vi "UI.vi"(8 "ErrorIn":errorcluster, 11 "QueuesIn":T1) -> (0 "ErrorOut":errorcluster, 3 "QueuesOut":T1)   [LabVIEW 2019]
uses:
  utilities/AQueues.ctl
  AmasterVIs/ACommand.ctl
  analyzeAccelerationDataVIs/AnalyzedVibrationsData.ctl
  analyzeAccelerationDataVIs/AccelerationDataFrames.ctl
  analyzeAccelerationDataVIs/calculateFaultIndicatorsVIs/FaultDetections.ctl
  analyzeAccelerationDataVIs/calculateFaultIndicatorsVIs/ParameterFaultDetection.ctl
  analyzeAccelerationDataVIs/calculateFaultIndicatorsVIs/FaultParameter.ctl
  analyzeAccelerationDataVIs/calculateFaultIndicatorsVIs/FrequencyFaultDetection.ctl
  analyzeAccelerationDataVIs/calculateFaultIndicatorsVIs/OrdersFaultDetection.ctl
  TDMSmanagerVIs/TDMSAnalyzerData.ctl
  TDMSmanagerVIs/TDMSAnalyzerDataType.ctl
  UIVIs/UIState.ctl
  <vilib>/dex/Stream Element Allocation Mode.ctl
  VibrationDiagnosisDesktopApp/mainVIs/communicateWithAnalyzerVIs/ReceiverData.ctl
  VibrationDiagnosisDesktopApp/mainVIs/communicateWithAnalyzerVIs/ReceiverDataType.ctl
  UIVIs/UIOutputFGVAction.ctl
  <vilib>/myRIO/Instrument Drivers/Onboard IO/DIO/typedefs/DIO Reference.ctl
  <vilib>/myRIO/Common/Instrument Driver Framework/Utilities/typedefs/myRIO Generic Hardware Reference.ctl
  <vilib>/myRIO/Common/Instrument Driver Framework/Utilities/typedefs/Hardware Version Enum.ctl
  <vilib>/myRIO/Common/Instrument Driver Framework/Utilities/typedefs/myRIO v1.0 Reference.ctl
  <vilib>/myRIO/Common/Instrument Driver Framework/Utilities/typedefs/Generic FPGA Reference.ctl
  <vilib>/myRIO/Common/Instrument Driver Framework/myRIO v1.0/DIO/typedefs/DIO Channels List.ctl
  <vilib>/myRIO/Common/Instrument Driver Framework/myRIO v1.0/DIO/typedefs/DIO Channels Enum.ctl
  <vilib>/userdefined/High Color/nirio_resource_hc.ctl
  VibrationDiagnosisDesktopApp/mainVIs/communicateWithAnalyzerVIs/SenderData.ctl
  VibrationDiagnosisDesktopApp/mainVIs/communicateWithAnalyzerVIs/SenderDataType.ctl
  utilities/FGVAction.ctl
  VibrationDiagnosisDesktopApp/mainVIs/DialogsVIs/AnalysisSettings.ctl
  analyzeAccelerationDataVIs/calculateFaultIndicatorsVIs/Thresholds.ctl
  aquireAccelerationDataVIs/Accelerometer.ctl
  <vilib>/myRIO/Common/Instrument Driver Framework/Utilities/vis/Is FPGA Ref Available.vi
  <vilib>/myRIO/Common/Instrument Driver Framework/myRIO v1.0/DIO/vis/myRIO v1.1 Open Throughput DIO.vi
  <vilib>/myRIO/Instrument Drivers/Onboard IO/DIO/vis/Read.vi
  <vilib>/myRIO/Instrument Drivers/Onboard IO/DIO/vis/Write.vi
  <vilib>/myRIO/Common/Instrument Driver Framework/Utilities/vis/Validate Channels.vi
  <vilib>/myRIO/Common/Instrument Driver Framework/myRIO v1.0/DIO/vis/myRIO v1.0 Reserve DIO.vi
  <vilib>/myRIO/Common/Instrument Driver Framework/myRIO v1.0/Resource Manager/vis/myRIO v1.0 Reserve Channel List.vi
  <vilib>/myRIO/Common/Instrument Driver Framework/myRIO v1.0/DIO/vis/myRIO v1.0 Build MUX Configuration DIO.vi
  <vilib>/myRIO/Common/Instrument Driver Framework/myRIO v1.0/Resource Manager/vis/myRIO v1.0 Reserve Channel.vi
  <vilib>/myRIO/Common/Instrument Driver Framework/myRIO v1.0/Resource Manager/vis/myRIO v1.0 Unreserve Channel.vi
  <vilib>/myRIO/Common/Instrument Driver Framework/myRIO v1.0/Resource Manager/vis/myRIO v1.0 Create Configuration List.vi
  <vilib>/myRIO/Common/Instrument Driver Framework/myRIO v1.0/Resource Manager/vis/myRIO v1.0 Build Mutex Name.vi
  <vilib>/Utility/VariantDataType/GetNumericInfo.vi
  <vilib>/Utility/error.llb/Error Cluster From Error Code.vi
  <vilib>/myRIO/Common/Instrument Driver Framework/myRIO v1.0/myRIO v1.1 Open Throughput.vi
  <vilib>/myRIO/Common/Instrument Driver Framework/Utilities/vis/IO Manager.vi
  <vilib>/myRIO/Common/Instrument Driver Framework/Utilities/vis/Configuration Manager.vi
  <vilib>/myRIO/Common/Instrument Driver Framework/myRIO v1.0/Resource Manager/vis/myRIO v1.0 Configure IO.vi
  <vilib>/myRIO/Common/Instrument Driver Framework/myRIO v1.0/myRIO v1.0 Close.vi
  <vilib>/myRIO/Common/Instrument Driver Framework/myRIO v1.0/DIO/vis/myRIO v1.0 Read DIO.vi
  <vilib>/myRIO/Common/Instrument Driver Framework/myRIO v1.0/DIO/vis/myRIO v1.0 Write DIO.vi
  <vilib>/myRIO/Express VI/Onboard Devices/Button/Button Express VI.xnode
  <vilib>/myRIO/Instrument Drivers/Onboard IO/DIO/vis/myRIO DIO Open.xnode
  <vilib>/myRIO/Express VI/Onboard Devices/LED/LED Express VI.xnode
  <vilib>/myRIO/Instrument Drivers/Onboard IO/DIO/DIO.lvlib
panel:
  in  "Restart":bool
  in  "OutputConnected":bool
  in  "InputConnected":bool
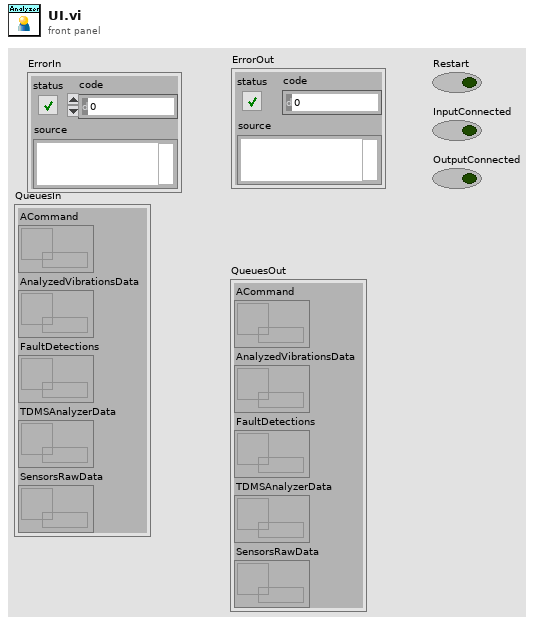
[diagram p1: front panel]
types:
  T1 = typedef "AQueues.ctl" = cluster{"ACommand":refnum<queue>, "AnalyzedVibrationsData":refnum<queue>, "FaultDetections":refnum<queue>, "TDMSAnalyzerData":refnum<queue>, "SensorsRawData":refnum<queue>}
  T2 = typedef "UIState.ctl" = enum16{"Connect", "Communicate", "Disconnect"}
  T3 = typedef "ACommand.ctl" = enum16{"None", "Start", "Stop", "Restart", "SendFilesData", "DeleteAllData", "ButtonClicked"}
  T4 = typedef "DIO.lvlib/DIO Reference.ctl" = cluster{"myRIO Reference":T5, "DIO Channels List":T9}
  T5 = typedef "myRIO Generic Hardware Reference.ctl" = cluster{"myRIO Model":T6, "myRIO Hardware Reference":T7}
  T6 = typedef "Hardware Version Enum.ctl" = enum16{"Unknown", "myRIO-1900", "myRIO-1950", "roboRIO", "NI ELVIS RIO CM", "ELVIS III"}
  T7 = typedef "myRIO v1.0 Reference.ctl" = cluster{"Generic FPGA Reference":T8, "Allow multiple opens":bool}
  T8 = typedef "Generic FPGA Reference.ctl" = refnum<k20>
  T9 = typedef "DIO Channels List.ctl" = T10[]
  T10 = typedef "DIO Channels Enum.ctl" = enum16{"Not Connected", "C/DIO0", "C/DIO1", "C/DIO2", "C/DIO3", "C/DIO4", "C/DIO5", "C/DIO6", "C/DIO7", "A/DIO0", "A/DIO1", "A/DIO2", "A/DIO3", "A/DIO4", "A/DIO5", "A/DIO6", "A/DIO7", "A/DIO8", "A/DIO9", "A/DIO10", "A/DIO11", "A/DIO12", "A/DIO13", "A/DIO14", "A/DIO15", "A/DIO16", "A/DIO17", "A/DIO18", "A/DIO19", "B/DIO0", "B/DIO1", "B/DIO2", "B/DIO3", "B/DIO4", "B/DIO5", "B/DIO6", "B/DIO7", "B/DIO8", "B/DIO9", "B/DIO10", "B/DIO11", "B/DIO12", "B/DIO13", "B/DIO14", "B/DIO15", "B/DIO16", "B/DIO17", "B/DIO18", "B/DIO19", "LED0", "LED1", "LED2", "LED3", "Button0", "DIO/DIO0", "DIO/DIO1", "DIO/DIO2", "DIO/DIO3", "DIO/DIO4", "DIO/DIO5", "DIO/DIO6", "DIO/DIO7", "DIO/DIO8", "DIO/DIO9", "SPI/CS0", "SPI/CS1", "SPI/CS2", "SPI/CS3", "LED RADIO (Green)", "LED RADIO (Red)", "LED COMM (Green)", "LED COMM (Red)", "LED MODE (Green)", "LED MODE (Red)"}
  T11 = typedef "nirio_resource_hc.ctl" = tag
  T12 = typedef "ReceiverData.ctl" = cluster{"ReceiverDataType":T13, "Data":string}
  T13 = typedef "ReceiverDataType.ctl" = enum16{"UIOutput", "AnalyzedVibrationsData", "TDMSFiles"}
  T14 = typedef "UIOutputFGVAction.ctl" = enum16{"Read", "Write", "CheckUpdate", "SetUpdated"}
  T15 = typedef "Stream Element Allocation Mode.ctl" = u32
  T16 = typedef "AnalyzerSettings.ctl" = cluster{"Create NS Timeout Code":i32, "Destroy NS Timeout Code":i32, "All threads":T17[], "Connected to app?":bool, "AnalysisSettings":T18}
  T17 = typedef "AThreads.ctl" = enum16{"UI", "analyzeAccelerationData", "aquireAccelerationData", "communicateWebServices", "TDMSmanager", "aquireTachoSignal"}
  T18 = typedef "AnalysisSettings.ctl" = cluster{"Fault Thresholds":T19, "Analysis series name":string, "Save data analysis?":bool, "Band size":i32, "OrderAnalysis?":bool, "Accelerometer":T21, "fs [Hz]":dbl, "Pulse per revolution":u16}
  T19 = typedef "Thresholds.ctl" = cluster{"Parameters labels":T20[], "Parameters thresholds":dbl[], "Freqs and thresholds":dbl[][], "Orders and thresholds":dbl[][]}
  T20 = typedef "FaultParameter.ctl" = enum16{"Kurtosis", "RMS", "Crest factor"}
  T21 = typedef "Accelerometer.ctl" = enum16{"None", "MPU6050", "MMA7351"}
  T22 = typedef "AnalyzedVibrationsData.ctl" = cluster{"AccelerationDataFrames":T23, "Fault detections":T24, "Order Power Spectra":cluster{"order 0":dbl, "delta order":dbl, "magnitude":dbl[]}[], "Tacho signal":waveform(dbl), "Rotational speed [RPM]":dbl}
  T23 = typedef "AccelerationDataFrames.ctl" = cluster{"AccelerationData":waveform(dbl)[], "Amplitudes":cluster{"f0":dbl, "df":dbl, "real part":dbl[]}[], "Phases":cluster{"f0":dbl, "df":dbl, "imaginary part":dbl[]}[]}
  T24 = typedef "FaultDetections.ctl" = cluster{"Parameters fault detection":T25[], "Frequencies fault detection":T26[], "Orders fault detection":T27[]}
  T25 = typedef "ParameterFaultDetection.ctl" = cluster{"Axes Values":dbl[], "Axes Fault Detection":bool[], "Parameter Label":T20}
  T26 = typedef "FrequencyFaultDetection.ctl" = cluster{"Axes Values":dbl[], "Axes Fault Detection":bool[], "Frequency":dbl}
  T27 = typedef "OrdersFaultDetection.ctl" = cluster{"Order":dbl, "Axes Fault Detection":bool[], "Axes Values":dbl[]}
  T28 = typedef "UIOutput.ctl" = cluster{"Aquiring data":bool, "AnalyzerError":errorcluster, "FIFO overflow":bool, "Analyzing data":bool}
  T29 = typedef "TDMSAnalyzerData.ctl" = cluster{"TDMSAnalyzerDataType":T30, "group name out":string, "channel name(s) out":string[], "data":waveform(dbl)[], "File name":string}
  T30 = typedef "TDMSAnalyzerDataType.ctl" = enum16{"FileDataStart", "FileGroup", "FileDataStop", "NewFile", "EndOfFile"}
  T31 = typedef "FGVAction.ctl" = enum16{"Read", "Write"}
  T32 = typedef "SenderData.ctl" = cluster{"SenderDataType":T33, "Data":string}
  T33 = typedef "SenderDataType.ctl" = enum16{"Command", "AnalysisSettings"}
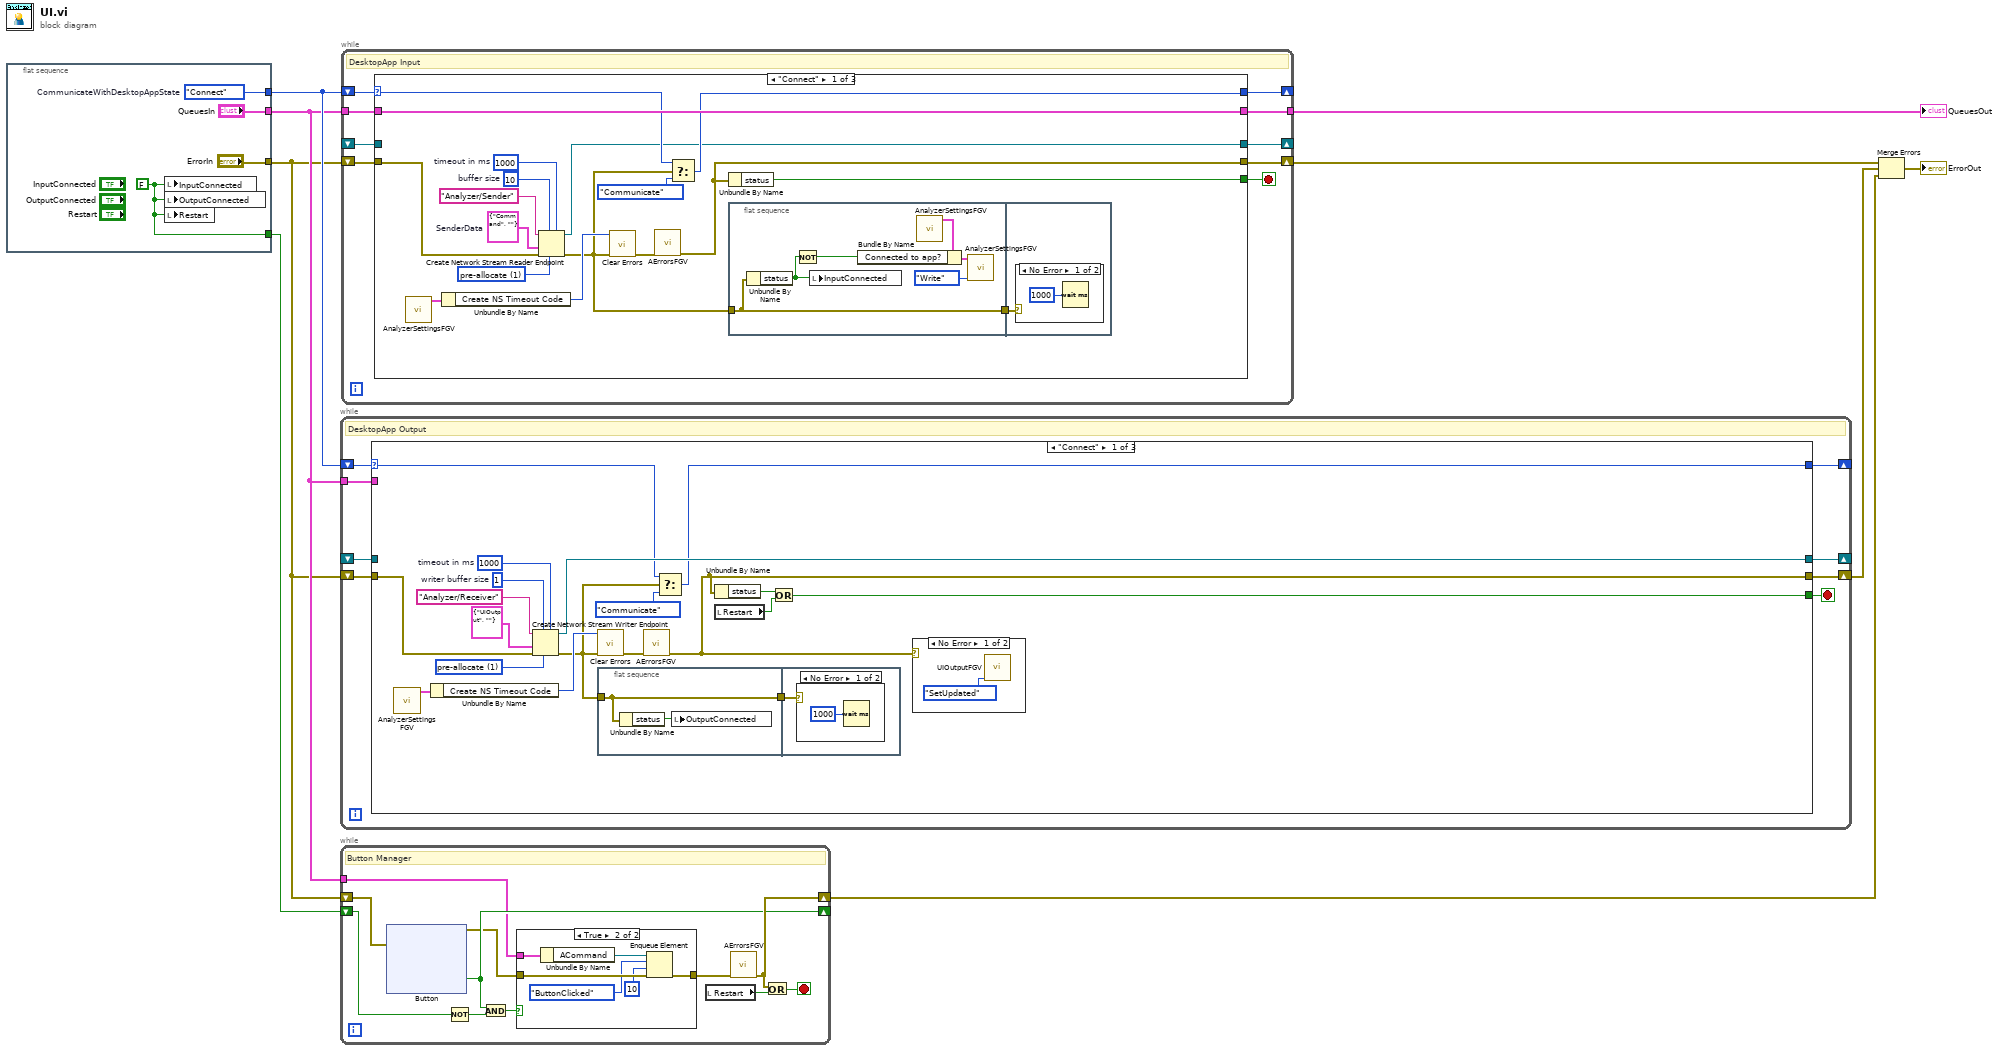
[diagram p0: block diagram]
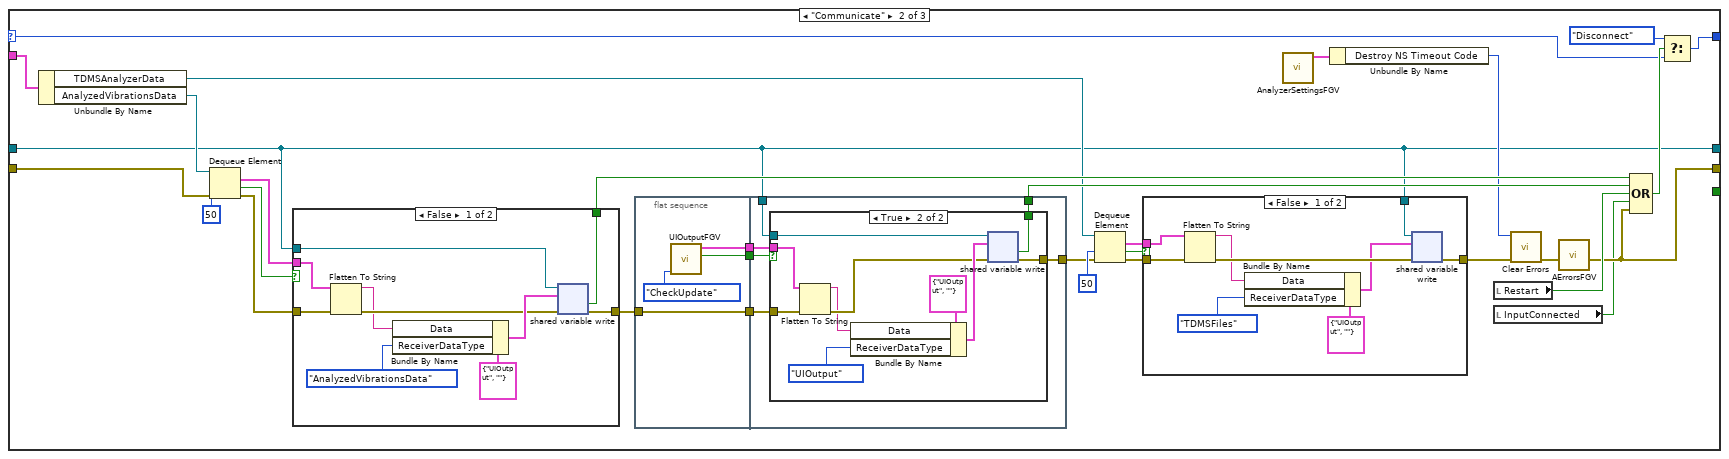
[diagram p5: hidden frame]
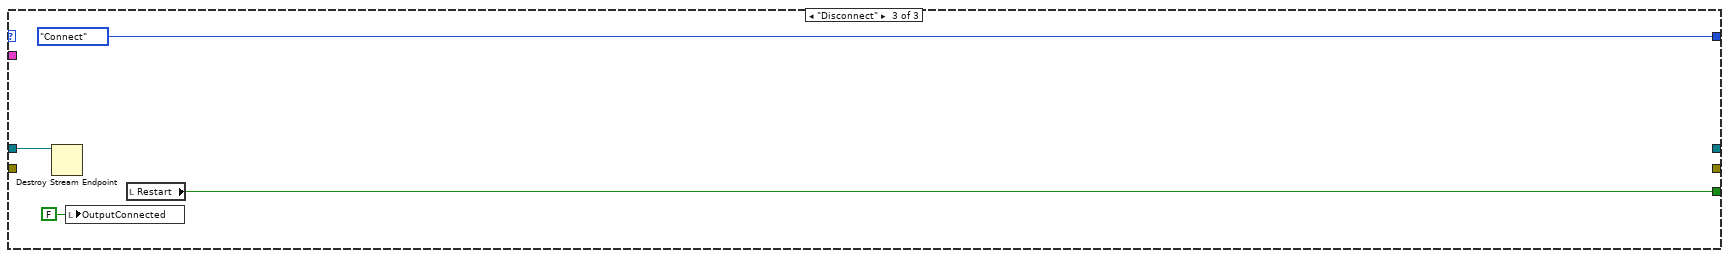
[diagram p9: hidden frame]
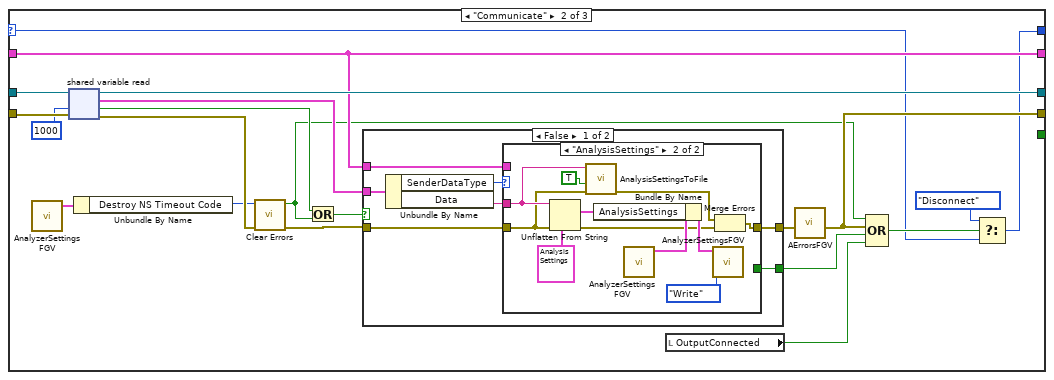
[diagram p11: hidden frame]
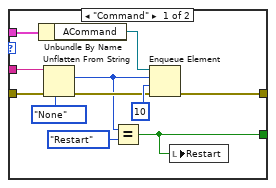
[diagram p12: hidden frame]
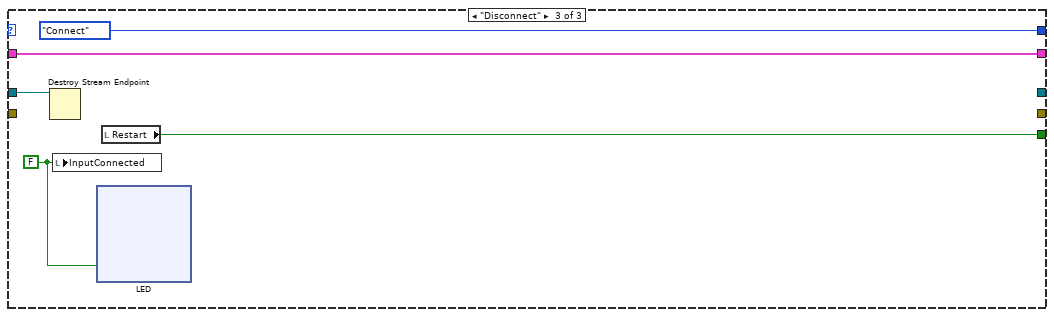
[diagram p14: hidden frame]
diagram:
  n1 = flat-sequence {
    tunnel: [w13] -> w9
    tunnel: ["QueuesIn"] -> w4
    tunnel: ["ErrorIn"] -> w3
    tunnel: [w10] -> w1
    frame #0 {
      w10 = FALSE ("InputConnected")
      w13 = UIState."Connect"  # CommunicateWithDesktopAppState
      n2 = local write "InputConnected"(w10) -> ()
      n3 = local write "OutputConnected"(w10) -> ()
      n4 = local write "Restart"(w10) -> ()
    }
  }
  n5 = while {
    tunnel: w4 -> [w16]
    shift-right: [w22] -> w2
    shift-left: w3 -> [w24]
    shift-right: [w20] -> _
    shift-left: w1 -> [w19]
    stop <- w21 stop-if-true
    # "Button Manager"
    n6 = xnode "Button"("error in (no error)"=w24) -> ("Value"=w20:bool, "error out"=w15:errorcluster)
    n7 = Not(x=w19) -> (.not. x?=w18:bool)
    n8 = And(x=w20, y=w18) -> (x .and. y?=w17:bool)
    n9 = case shown="True" w17 {
      tunnel: w16 -> [_ w31]
      tunnel: w15 -> [w25 w29]
      tunnel: [w25 w26] -> w14
      frame False {
      }
      frame True {
        n10 = Unbundle By Name(w31) -> ("ACommand"=w30:refnum<queue>)
        n11 = Enqueue Element(queue=w30, element=ACommand."ButtonClicked", timeout in ms (-1)=10, error in (no error)=w29) -> (error out=w26:errorcluster)  [unwired: 2 out]
      }
    }
    n12 = local read "Restart"() -> (w23:bool)
    n13 = call "AErrorsFGV.vi"("CriticalErrorIn"=w14) -> ("CriticalErrorOut"=w22:errorcluster)  [unwired: 7 in, 3 out]
    n14 = Or(x=w22, y=w23) -> (x .or. y?=w21:bool)
  }
  n15 = while {
    shift-right: [w68] -> _
    shift-left: w9 -> [w74]
    tunnel: w4 -> [w73]
    shift-right: [w70] -> w6
    shift-left: w3 -> [w72]
    shift-right: [w71] -> _
    shift-left: _ -> [w67]
    stop <- w69 stop-if-true
    # "DesktopApp Output"
    n16 = case shown="\"Connect\"" w74 {
      selector: w74 -> [w80 w116 _]
      tunnel: w73 -> [_ w129 _]
      tunnel: w72 -> [w88 w128 _]
      tunnel: [w87 w99 _] -> w71
      tunnel: [w75 w112 _] -> w70
      tunnel: [w76 _ w172] -> w69
      tunnel: [w79 w114 UIState."Connect" ("CommunicateWithDesktopAppState")] -> w68
      tunnel: w67 -> [_ w99 w174]
      frame "Connect" {
        w92 = T15 1 items=["allocate as needed", "pre-allocate"] ("element allocation mode")
        w93 = 1000  # timeout in ms
        w91 = 1  # writer buffer size
        n17 = call "AnalyzerSettingsFGV.vi"() -> ("AnalyzerSettingsOut"=w85:T16)  [unwired: 11 in]
        n18 = Unbundle By Name(w85) -> ("Create NS Timeout Code"=w84:i32)
        n19 = Create Network Stream Writer Endpoint(5:w93, 6:w92, 7:w91, 8:w88, 9:T12 {"ReceiverDataType"=enum."UIOutput", "Data"=""} ("ReceiverData"), 11:"Analyzer/Receiver" ("writer name")) -> (0:w81:errorcluster, 3:w87:refnum<k21>)  [unwired: 1 in]
        n20 = call <vilib>:"Clear Errors.vi"("error in (no error)"=w81, "specific error code to clear (0: all)"=w84) -> ("error out"=w86:errorcluster)  [unwired: 4 in, 1 out]
        n21 = flat-sequence {
          tunnel: w81 -> [w96]
          tunnel: [w96] -> w82
          tunnel: w82 -> [w97]
          frame #0 {
            n22 = Unbundle By Name(w96) -> ("status"=w95:bool)
            n23 = local write "OutputConnected"(w95) -> ()
          }
          frame #1 {
            n24 = case shown="No Error" w97 {
              frame No Error {
                n25 = Wait (ms)(milliseconds to wait=u32 1000) -> ()  [unwired: 1 out]
              }
              frame Error {
              }
            }
          }
        }
        n26 = call "AErrorsFGV.vi"("CriticalErrorIn"=w86) -> ("CriticalErrorOut"=w75:errorcluster)  [unwired: 7 in, 3 out]
        n27 = Select(t=w80, s=w81, f=UIState."Communicate" ("t")) -> (s? t:f=w79:T2)
        n28 = Unbundle By Name(w75) -> ("status"=w77:bool)
        n29 = local read "Restart"() -> (w78:bool)
        n30 = Or(x=w77, y=w78) -> (x .or. y?=w76:bool)
        n31 = case shown="No Error" w75 {
          frame No Error {
            n32 = call "UIOutputFGV.vi"("FGVAction (Read)"=UIOutputFGVAction."SetUpdated") -> ()  [unwired: 9 in, 2 out]
          }
          frame Error {
          }
        }
      }
      frame "Communicate" {
        n33 = Unbundle By Name(w129) -> ("TDMSAnalyzerData"=w104:refnum<queue>, "AnalyzedVibrationsData"=w107:refnum<queue>)
        n34 = Dequeue Element(queue=w107, timeout in ms (-1)=50, error in (no error)=w128) -> (element=w124:T22, timed out?=w126:bool, error out=w125:errorcluster)  [unwired: 1 out]
        n35 = case shown="False" w126 {
          tunnel: w125 -> [w165 w171]
          tunnel: w124 -> [w163 _]
          tunnel: w99 -> [w170 _]
          tunnel: [w168 w171] -> w122
          tunnel: [w166 _] -> w119
          frame False {
            n36 = Flatten To String(anything=w163, error in (no error)=w165) -> (data string=w161:string, error out=w164:errorcluster)  [unwired: 2 in, 1 out]
            n37 = Bundle By Name(cluster=T12 {"ReceiverDataType"=enum."UIOutput", "Data"=""} ("data in"), "Data"=w161, "ReceiverDataType"=ReceiverDataType."AnalyzedVibrationsData") -> (w167:T12)
            n38 = shared-variable-write(w170, w164, w167) -> (w168:errorcluster, w166:bool)  [unwired: 1 in, 1 out]
          }
          frame True {
          }
        }
        n39 = flat-sequence {
          tunnel: [w142] -> w123
          tunnel: w122 -> [w141]
          tunnel: [w141] -> w121
          tunnel: [w140] -> w120
          tunnel: w123 -> [w149]
          tunnel: w121 -> [w147]
          tunnel: w120 -> [w148]
          tunnel: w99 -> [w146]
          tunnel: [w145] -> w105
          tunnel: [w144] -> w118
          frame #0 {
            n40 = call "UIOutputFGV.vi"("FGVAction (Read)"=UIOutputFGVAction."CheckUpdate") -> ("Updated?"=w142:bool, "UIOutputOut"=w140:T28)  [unwired: 9 in]
          }
          frame #1 {
            n41 = case shown="True" w149 {
              tunnel: w148 -> [_ w153]
              tunnel: w147 -> [w150 w155]
              tunnel: w146 -> [_ w160]
              tunnel: [w150 w157] -> w145
              tunnel: [_ w156] -> w144
              frame False {
              }
              frame True {
                n42 = Flatten To String(anything=w153, error in (no error)=w155) -> (data string=w152:string, error out=w154:errorcluster)  [unwired: 2 in, 1 out]
                n43 = Bundle By Name(cluster=T12 {"ReceiverDataType"=enum."UIOutput", "Data"=""} ("data in"), "Data"=w152, "ReceiverDataType"=ReceiverDataType."UIOutput") -> (w158:T12)
                n44 = shared-variable-write(w160, w154, w158) -> (w157:errorcluster, w156:bool)  [unwired: 1 in, 1 out]
              }
            }
          }
        }
        n45 = Dequeue Element(queue=w104, timeout in ms (-1)=50, error in (no error)=w105) -> (element=w102:T29, timed out?=w103:bool, error out=w101:errorcluster)  [unwired: 1 out]
        n46 = case shown="False" w103 {
          tunnel: w102 -> [w134 _]
          tunnel: w101 -> [w133 w139]
          tunnel: [w130 w139] -> w100
          tunnel: w99 -> [w131 _]
          frame False {
            n47 = Flatten To String(anything=w134, error in (no error)=w133) -> (data string=w136:string, error out=w137:errorcluster)  [unwired: 2 in, 1 out]
            n48 = Bundle By Name(cluster=T12 {"ReceiverDataType"=enum."UIOutput", "Data"=""} ("data in"), "Data"=w136, "ReceiverDataType"=ReceiverDataType."TDMSFiles") -> (w132:T12)
            n49 = shared-variable-write(w131, w137, w132) -> (w130:errorcluster)  [unwired: 1 in, 2 out]
          }
          frame True {
          }
        }
        n50 = call "AnalyzerSettingsFGV.vi"() -> ("AnalyzerSettingsOut"=w110:T16)  [unwired: 11 in]
        n51 = Unbundle By Name(w110) -> ("Destroy NS Timeout Code"=w108:i32)
        n52 = local read "Restart"() -> (w113:bool)
        n53 = local read "InputConnected"() -> (w111:bool)
        n54 = call <vilib>:"Clear Errors.vi"("error in (no error)"=w100, "specific error code to clear (0: all)"=w108) -> ("error out"=w109:errorcluster)  [unwired: 4 in, 1 out]
        n55 = call "AErrorsFGV.vi"("InternalErrorIn"=w109) -> ("InternalErrorOut"=w112:errorcluster)  [unwired: 7 in, 3 out]
        n56 = Compound Arithmetic op=OR(w119, w118, w113, w111, w112) -> (w117:bool)
        n57 = Select(t=UIState."Disconnect", s=w117, f=w116) -> (s? t:f=w114:T2)
      }
      frame "Disconnect" {
        n58 = Destroy Stream Endpoint(11:w174) -> ()  [unwired: 1 in, 1 out]
        n59 = local write "OutputConnected"(FALSE ("OutputConnected")) -> ()
        n60 = local read "Restart"() -> (w172:bool)
      }
    }
  }
  n61 = while {
    tunnel: w4 -> [w180]
    shift-right: [w178] -> _
    shift-left: w9 -> [w184]
    shift-right: [w177] -> _
    shift-left: _ -> [w176]
    shift-right: [w183] -> w7
    shift-left: w3 -> [w182]
    tunnel: [w179] -> w8
    stop <- w181 stop-if-true
    # "DesktopApp Input"
    n62 = case shown="\"Connect\"" w184 {
      selector: w184 -> [w190 w220 _]
      tunnel: [w192 w224 _] -> w183
      tunnel: w182 -> [w194 w229 _]
      tunnel: [w191 _ w263] -> w181
      tunnel: w180 -> [w202 w227 w265]
      tunnel: [w202 w227 w265] -> w179
      tunnel: [w193 w218 UIState."Connect" ("CommunicateWithDesktopAppState")] -> w178
      tunnel: [w188 w230 _] -> w177
      tunnel: w176 -> [_ w231 w264]
      frame "Connect" {
        w185 = T32 {"SenderDataType"=enum."Command", "Data"=""}  # SenderData
        w198 = 1000  # timeout in ms
        w197 = T15 1 items=["allocate as needed", "pre-allocate"] ("element allocation mode")
        w196 = 10  # buffer size
        n63 = call "AnalyzerSettingsFGV.vi"() -> ("AnalyzerSettingsOut"=w199:T16)  [unwired: 11 in]
        n64 = Unbundle By Name(w199) -> ("Create NS Timeout Code"=w200:i32)
        n65 = Create Network Stream Reader Endpoint(5:w198, 6:w197, 7:w196, 8:w194, 9:w185, 11:"Analyzer/Sender" ("reader name")) -> (0:w187:errorcluster, 3:w188:refnum<k21>)  [unwired: 1 in]
        n66 = call <vilib>:"Clear Errors.vi"("error in (no error)"=w187, "specific error code to clear (0: all)"=w200) -> ("error out"=w201:errorcluster)  [unwired: 4 in, 1 out]
        n67 = call "AErrorsFGV.vi"("CriticalErrorIn"=w201) -> ("CriticalErrorOut"=w192:errorcluster)  [unwired: 7 in, 3 out]
        n68 = Select(t=w190, s=w187, f=UIState."Communicate" ("t")) -> (s? t:f=w193:T2)
        n69 = Unbundle By Name(w192) -> ("status"=w191:bool)
        n70 = flat-sequence {
          tunnel: w187 -> [w208]
          tunnel: [w208] -> w186
          tunnel: w186 -> [w209]
          frame #0 {
            n71 = Unbundle By Name(w208) -> ("status"=w207:bool)
            n72 = Not(x=w207) -> (.not. x?=w203:bool)
            n73 = local write "InputConnected"(w207) -> ()
            n74 = call "AnalyzerSettingsFGV.vi"() -> ("AnalyzerSettingsOut"=w204:T16)  [unwired: 11 in]
            n75 = Bundle By Name(cluster=w204, "Connected to app?"=w203) -> (w206:T16)
            n76 = call "AnalyzerSettingsFGV.vi"("FGVAction (Read)"=FGVAction."Write", "AnalyzerSettingsIn"=w206) -> ()  [unwired: 9 in, 1 out]
          }
          frame #1 {
            n77 = case shown="No Error" w209 {
              frame No Error {
                n78 = Wait (ms)(milliseconds to wait=u32 1000) -> ()  [unwired: 1 out]
              }
              frame Error {
              }
            }
          }
        }
      }
      frame "Communicate" {
        n79 = call "AnalyzerSettingsFGV.vi"() -> ("AnalyzerSettingsOut"=w217:T16)  [unwired: 11 in]
        n80 = shared-variable-read(w231, w229, 1000 ("timeout ms (-1)")) -> (w230:refnum<k21>, w216:errorcluster, w212:bool, w226:T32)
        n81 = Unbundle By Name(w217) -> ("Destroy NS Timeout Code"=w214:i32)
        n82 = call <vilib>:"Clear Errors.vi"("error in (no error)"=w216, "specific error code to clear (0: all)"=w214) -> ("error out"=w215:errorcluster, "specific error cleared?"=w211:bool)  [unwired: 4 in]
        n83 = Or(x=w212, y=w211) -> (x .or. y?=w213:bool)
        n84 = case shown="False" w213 {
          tunnel: w227 -> [w238 _]
          tunnel: w226 -> [w234 _]
          tunnel: w215 -> [w237 w261]
          tunnel: [w236 w261] -> w225
          tunnel: [w235 _] -> w222
          frame False {
            n85 = Unbundle By Name(w234) -> ("SenderDataType"=w233:T33, "Data"=w232:string)
            n86 = case shown="\"AnalysisSettings\"" w233 {
              tunnel: w238 -> [w249 _]
              tunnel: w237 -> [w242 w254]
              tunnel: [w246 w253] -> w236
              tunnel: [w244 _] -> w235
              tunnel: w232 -> [w243 w257]
              frame "Command" {
                n87 = Unbundle By Name(w249) -> ("ACommand"=w248:refnum<queue>)
                n88 = Unflatten From String(type=ACommand."None" ("y"), binary string=w243, error in (no error)=w242) -> (value=w239:T3, error out=w241:errorcluster)  [unwired: 2 in, 1 out]
                n89 = Equal?(x=w239, y=ACommand."Restart") -> (x = y?=w244:bool)
                n90 = Enqueue Element(queue=w248, element=w239, timeout in ms (-1)=10, error in (no error)=w241) -> (error out=w246:errorcluster)  [unwired: 2 out]
                n91 = local write "Restart"(w244) -> ()
              }
              frame "AnalysisSettings" {
                n92 = Unflatten From String(type=T18 {"Fault Thresholds"={"Parameters labels"=[], "Parameters thresholds"=[], "Freqs and thresholds"=[], "Orders and thresholds"=[]}, "Analysis series name"="Analiza", "Save data analysis?"=TRUE, "Band size"=20, "OrderAnalysis?"=TRUE, "Accelerometer"=enum."MMA7351", "fs [Hz]"=4000.0, "Pulse per revolution"=1} ("AnalysisSettings"), binary string=w257, error in (no error)=w254) -> (value=w251:T18, error out=w255:errorcluster)  [unwired: 2 in, 1 out]
                n93 = call "AnalysisSettingsToFile.vi"("ErrorIn"=w254, "Save to file?"=TRUE, "AnalysisSettingsString"=w257) -> ("ErrorOut"=w252:errorcluster)  [unwired: 8 in]
                n94 = call "AnalyzerSettingsFGV.vi"() -> ("AnalyzerSettingsOut"=w260:T16)  [unwired: 11 in]
                n95 = Bundle By Name(cluster=w260, "AnalysisSettings"=w251) -> (w259:T16)
                n96 = call "AnalyzerSettingsFGV.vi"("FGVAction (Read)"=FGVAction."Write", "AnalyzerSettingsIn"=w259) -> ()  [unwired: 9 in, 1 out]
                n97 = Merge Errors(w252, w255) -> (w253:errorcluster)
              }
            }
          }
          frame True {
          }
        }
        n98 = local read "OutputConnected"() -> (w223:bool)
        n99 = call "AErrorsFGV.vi"("InternalErrorIn"=w225) -> ("InternalErrorOut"=w224:errorcluster)  [unwired: 7 in, 3 out]
        n100 = Compound Arithmetic op=OR(w211, w224, w222, w223) -> (w221:bool)
        n101 = Select(t=UIState."Disconnect", s=w221, f=w220) -> (s? t:f=w218:T2)
      }
      frame "Disconnect" {
        w262 = FALSE ("InputConnected")
        n102 = Destroy Stream Endpoint(11:w264) -> ()  [unwired: 1 in, 1 out]
        n103 = local write "InputConnected"(w262) -> ()
        n104 = xnode "LED"("LED0"=w262) -> ()  [unwired: 1 in, 1 out]
        n105 = local read "Restart"() -> (w263:bool)
      }
    }
  }
  "QueuesOut" <- w8
  n106 = Merge Errors(w7, w6, w2) -> (→"ErrorOut":errorcluster)
